vi "ERD_Read_List_Builder.vi"(0 "Array":T2(array[cluster]) {"ERD Number" format="%.0x"}, 5 "Error In":errorcluster) -> (14 "Read ERD List":T1[](array[typedef]) {"ERD Number" format="%.0x"}, 16 "ERD Name":string[](array[string]), 19 "Error Out":errorcluster)   [LabVIEW 2021]
doc: "This VI takes an array of ERD Cluster Data. Cluster conatins a boolean to Read the ERD or not, ERD number, name, and data type. It the compiles an array of ERD data to use in ERD Read VI."
uses:
  Common/LabVIEW GEA2 Toolkit/GEA3/type defs/ERD Read Data In.ctl
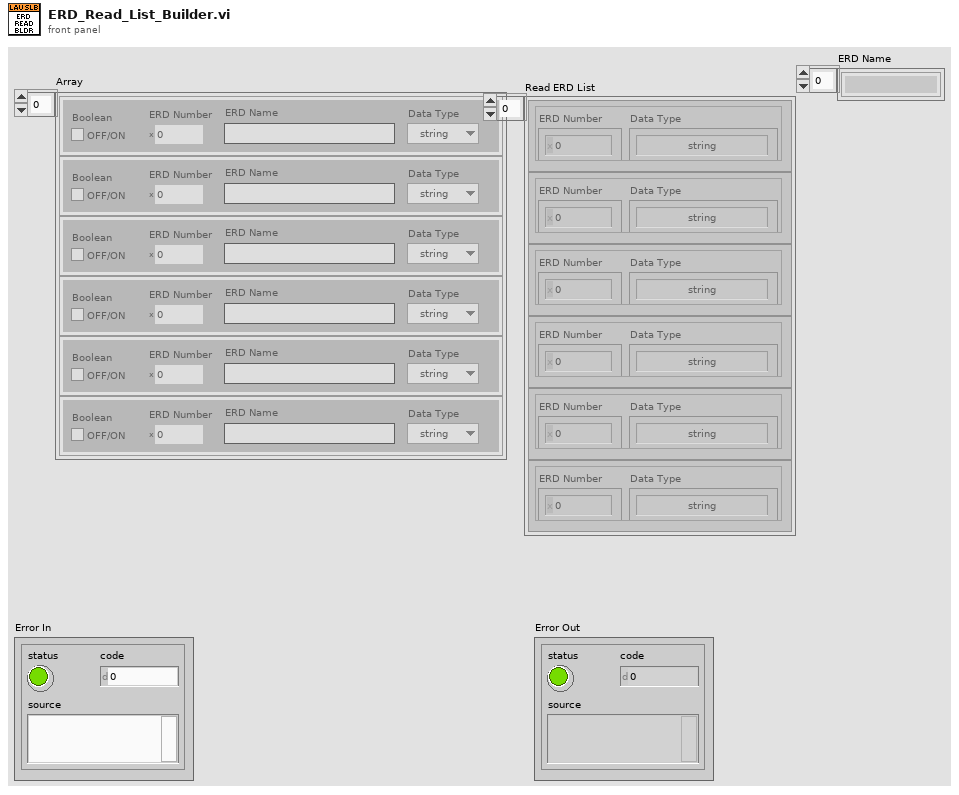
[diagram p1: front panel]
types:
  T1 = typedef "ERD Read Data In.ctl" = cluster{"ERD Number":u16, "Data Type":enum16{"string", "boolean", "uint8_t", "uint16_t", "uint32_t", "uint64_t", "int8_t", "int16_t", "int32_t", "int64_t"}}
  T2 = cluster{"Boolean":bool, "ERD Number":u16, "ERD Name":string, "Data Type":enum16{"string", "boolean", "uint8_t", "uint16_t", "uint32_t", "uint64_t"}}[]
  T3 = enum16{"string", "boolean", "uint8_t", "uint16_t", "uint32_t", "uint64_t"}
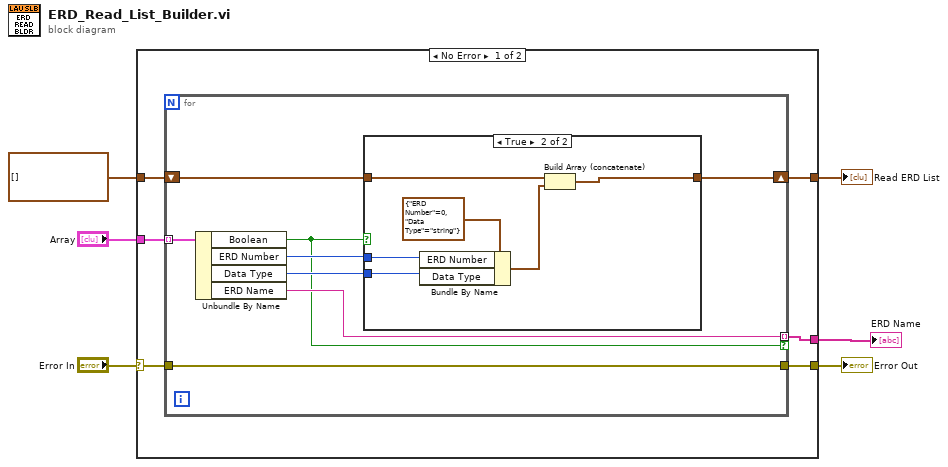
[diagram p0: block diagram]
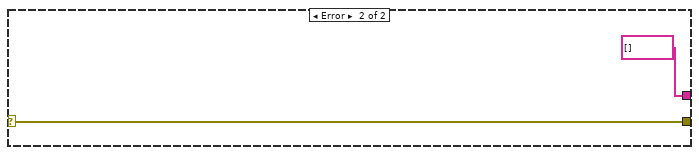
[diagram p3: hidden frame]
diagram:
  n1 = case shown="No Error" "Error In" {
    selector: "Error In" -> [w9 w29]
    tunnel: "Array" -> [w12 _]
    tunnel: [w11 _] -> w5
    tunnel: T1[] [] -> [w10 _]
    tunnel: [w8 w29] -> w2
    tunnel: [w7 string[] []] -> w1
    frame No Error {
      n2 = for {
        tunnel: w12 -> [w20] mode=indexing
        shift-right: [w17] -> w11
        shift-left: w10 -> [w18]
        tunnel: w9 -> [w15]
        tunnel: [w15] -> w8
        tunnel: [w14] -> w7 mode=indexing if=w13
        n3 = Unbundle By Name(w20) -> ("Boolean"=w13:bool, "ERD Number"=w19:u16, "Data Type"=w16:T3, "ERD Name"=w14:string)
        n4 = case shown="True" w13 {
          tunnel: w19 -> [_ w22]
          tunnel: w18 -> [w21 w27]
          tunnel: [w21 w25] -> w17
          tunnel: w16 -> [_ w23]
          frame False {
          }
          frame True {
            n5 = Bundle By Name(cluster=T1 {"ERD Number"=0, "Data Type"=enum."string"} ("ERD Read Data In"), "ERD Number"=w22, "Data Type"=w23) -> (w26:T1)
            n6 = Build Array (concatenate)(w27, w26) -> (w25:T1[])
          }
        }
      }
    }
    frame Error {
    }
  }
  "Read ERD List" <- w5
  "Error Out" <- w2
  "ERD Name" <- w1
